vi "Initialize.vi"(8 "error in (no error)":errorcluster, 11 "Sub Panel Actor in":refnum<class "Sub Panel Actor.lvclass">) -> (0 "error out":errorcluster, 3 "Sub Panel Actor out":refnum<class "Sub Panel Actor.lvclass">)   [LabVIEW 2020, in "Sub Panel Actor.lvlib" / "Sub Panel Actor.lvclass"]
uses:
  Sub Panel Actor.lvclass
  Sub Panel Actor.lvclass/Sub Panel Actor.ctl
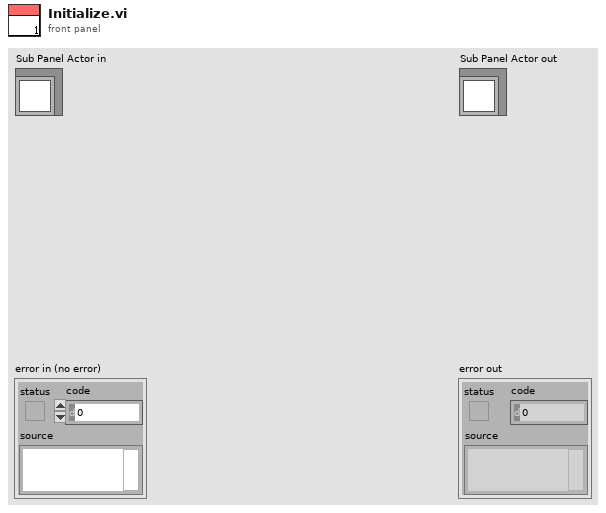
[diagram p1: front panel]
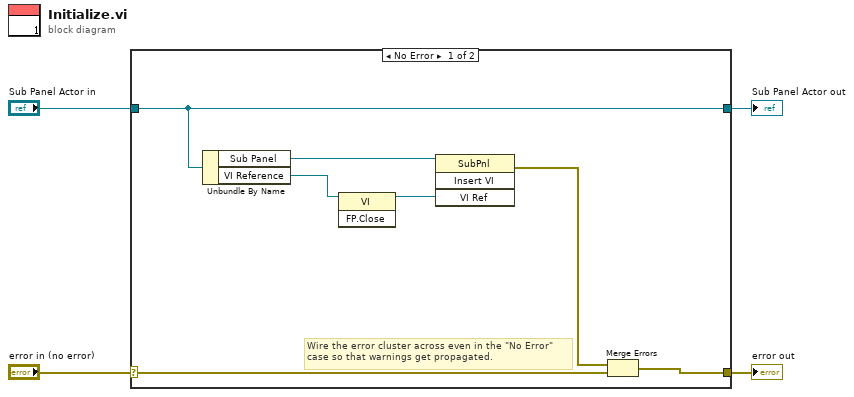
[diagram p0: block diagram]
diagram:
  n1 = case shown="No Error" "error in (no error)" {
    selector: "error in (no error)" -> [w11 w13]
    tunnel: [w6 w13] -> w3
    tunnel: [w10 w12] -> w1
    tunnel: "Sub Panel Actor in" -> [w10 w12]
    frame No Error {
      # "Wire the error cluster across even in the \"No Error\"\ncase so that warnings get propagated."
      n2 = Unbundle By Name(w10) -> ("Sub Panel"=w9:refnum<vi>, "VI Reference"=w8:refnum<vi>)
      n3 = invoke class="VI" method="FP.Close"(reference=w8) -> (reference out=w7:refnum<vi>)  [unwired: 2 in, 2 out]
      n4 = invoke class="SubPnl" method="Insert VI"(reference=w9, "VI Ref"=w7) -> (error out=w5:errorcluster)  [unwired: 2 in, 3 out]
      n5 = Merge Errors(w5, w11) -> (w6:errorcluster)
    }
    frame Error {
    }
  }
  "error out" <- w3
  "Sub Panel Actor out" <- w1
